vi "LAClear.vi"(8 "Error Input":errorcluster, 11 "LiteAgent In":T1) -> (0 "Error Output":errorcluster, 3 "LiteAgent Out":T1)   [LabVIEW 2017, in "LiteAgentSDK.lvlib"]
uses:
  LiteAgentSDK.lvlib
  C:/Users/Jan/Projects/LiteAgentSDK-LabVIEW/Source/Bin/LiteAgentSDK.LabVIEW.dll
  Bin/LiteAgentSDK.LabVIEW.dll
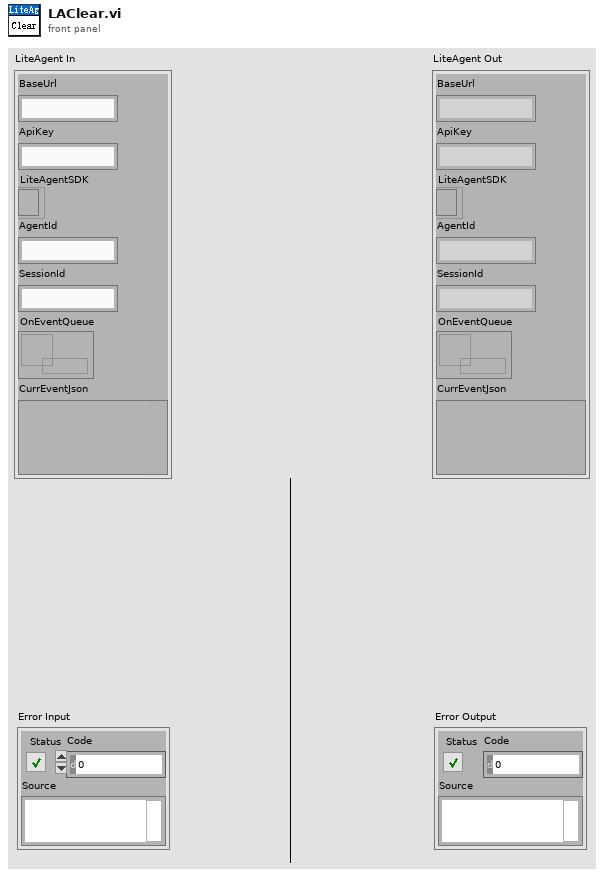
[diagram p1: front panel]
types:
  T1 = cluster{"BaseUrl":string, "ApiKey":string, "LiteAgentSDK":refnum<k24>, "AgentId":string, "SessionId":string, "OnEventQueue":refnum<queue>, "CurrEventJson":variant}
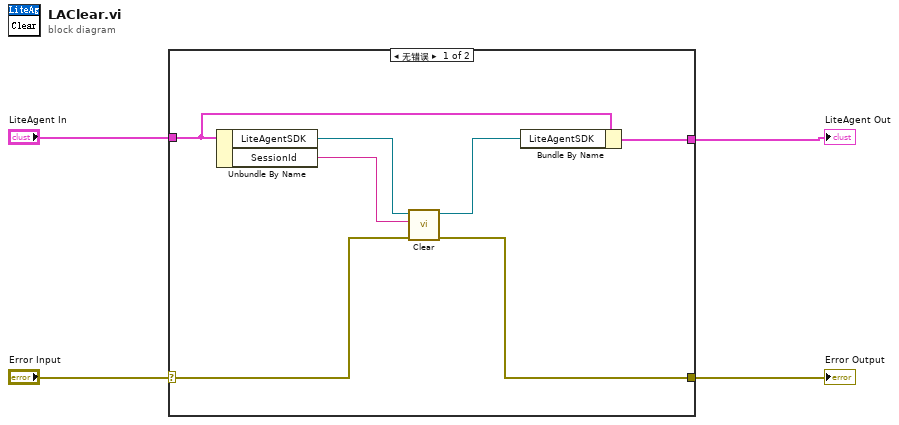
[diagram p0: block diagram]
diagram:
  n1 = case shown="无错误" "Error Input" {
    selector: "Error Input" -> [w11 w13]
    tunnel: [w10 w13] -> w3
    tunnel: "LiteAgent In" -> [w9 w12]
    tunnel: [w8 w12] -> w1
    frame No Error {
      n2 = Unbundle By Name(w9) -> ("LiteAgentSDK"=w7:refnum<k24>, "SessionId"=w5:string)
      n3 = call "Clear.vi"("Error Input"=w11, "SessionId"=w5, "LiteAgentSDK Input"=w7) -> ("Error Output"=w10:errorcluster, "LiteAgentSDK Output"=w6:refnum<k24>)  [unwired: 7 in]
      n4 = Bundle By Name(cluster=w9, "LiteAgentSDK"=w6) -> (w8:T1)
    }
    frame Error {
    }
  }
  "Error Output" <- w3
  "LiteAgent Out" <- w1
